vi "ResetTree.vi"(8 "Error In":errorcluster, 11 "Table in":refnum<vi>) -> (0 "Error Out":errorcluster)   [LabVIEW 2017, in "Client.lvlib" / "UI_API.lvlib"]
uses:
  UI_API.lvlib
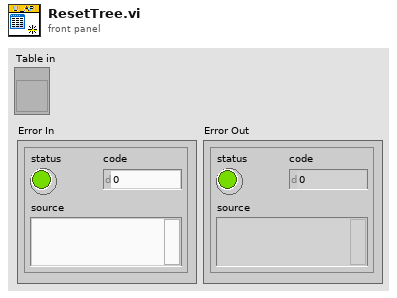
[diagram p1: front panel]
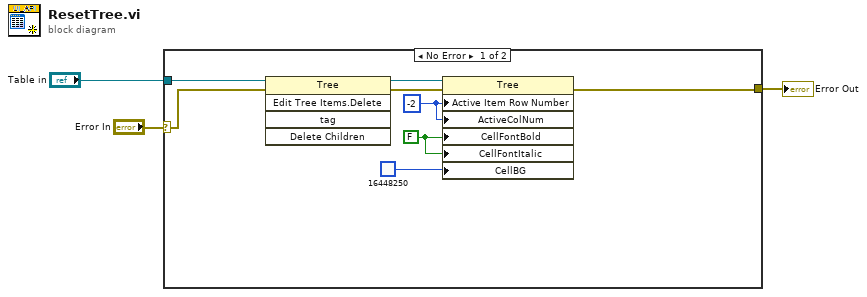
[diagram p0: block diagram]
diagram:
  n1 = case shown="No Error" "Error In" {
    selector: "Error In" -> [w7 w12]
    tunnel: "Table in" -> [w8 _]
    tunnel: [w4 w12] -> w1
    frame No Error {
      w11 = -2 ("Column")
      w10 = FALSE ("Active Cell:Cell Font:Italic")
      n2 = invoke on="Invoke Node" class="Tree" method="Edit Tree Items.Delete"(reference=w8, error in=w7) -> (reference out=w5:refnum<vi>, error out=w6:errorcluster)  [unwired: 3 in, 3 out]
      n3 = property on="Property Node" class="Tree"(reference=w5, error in=w6, "Active Item Row Number"=w11, "ActiveColNum"=w11, "CellFontBold"=w10, "CellFontItalic"=w10, "CellBG"=u32 16448250) -> (error out=w4:errorcluster)  [unwired: 1 out]
    }
    frame Error {
    }
  }
  "Error Out" <- w1
